vi "NS3_Msg.vi"(8 "error in":errorcluster, 11 "Msg":T1=enum."Exit") -> (0 "error out":errorcluster)   [LabVIEW 2010]
doc: "This VI implements the routine for sending messages to the NS3 actor. This routine gets the queue of the NS3 actor and sends an \"exit\" actor to the actor.\n\nCreated by Davis Montenegro\n06-23-2017"
uses:
  Ctrls/NS3_commands.ctl
  Vars/Comm_Vars.vi
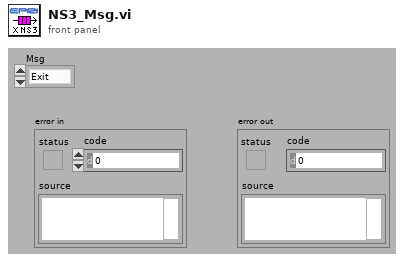
[diagram p1: front panel]
types:
  T1 = typedef "NS3_commands.ctl" = enum16{"Init NS3 Sim", "Step in", "Exit"}
  T2 = cluster{"actor_name":string, "actor_type":string, "queue":variant}[]
  T3 = cluster{"actor_name":string, "actor_type":string, "queue":variant}
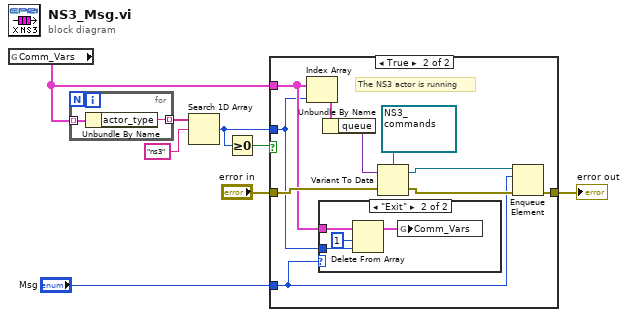
[diagram p0: block diagram]
diagram:
  n1 = global read "Comm_Vars.vi" "Comm_Vars"() -> (w3:T2)
  n2 = for {
    tunnel: w3 -> [w10] mode=indexing
    tunnel: [w9] -> w5 mode=indexing
    n3 = Unbundle By Name(w10) -> ("actor_type"=w9:string)
  }
  n4 = Search 1D Array(1D array=w5, element="ns3") -> (index of element=w2:i32)  [unwired: 1 in]
  n5 = Greater Or Equal To 0?(x=w2) -> (x >= 0?=w1:bool)
  n6 = case shown="True" w1 {
    tunnel: [w11 w20] -> w8
    tunnel: "error in" -> [w11 w18]
    tunnel: "Msg" -> [_ w14]
    tunnel: w3 -> [_ w13]
    tunnel: w2 -> [_ w12]
    frame False {
      # "The NS3 actor is not running, action cancelled"
    }
    frame True {
      w17 = refnum<queue> refnum items=["Init NS3 Sim", "Step in", "Exit"] ("queue")
      # "The NS3 actor is running"
      n7 = Index Array(array=w13, index=w12) -> (element=w15:T3)
      n8 = case shown="\"Exit\"" w14 {
        tunnel: w13 -> [_ w25]
        tunnel: w12 -> [_ w24]
        frame "Init NS3 Sim", Default {
        }
        frame "Exit" {
          n9 = Delete From Array(array=w25, length=1, index=w24) -> (array with subset deleted=w22:T2)  [unwired: 1 out]
          n10 = global write "Comm_Vars.vi" "Comm_Vars"(w22) -> ()
        }
      }
      n11 = Unbundle By Name(w15) -> ("queue"=w16:variant)
      n12 = Variant To Data(error in=w18, Variant=w16, type=w17) -> (error out=w19:errorcluster, data=w21:refnum<queue>)
      n13 = Enqueue Element(queue=w21, element=w14, error in (no error)=w19) -> (error out=w20:errorcluster)  [unwired: 1 in, 2 out]
    }
  }
  "error out" <- w8
